vi "Supported Typedefs FGV.vi"() -> (3 "supported typedefs":set{string}(c389))   [LabVIEW 2020, in "MeasurementLink Measurement Server.lvlib"]
uses:
  MeasurementLink Measurement Server.lvlib
  gRPC/Generated APIs/ni/protobuf/types/RPC Messages/ni_protobuf_types_DoubleXYData.ctl
  gRPC/Generated APIs/ni/protobuf/types/ni.protobuf.types.lvlib
  <vilib>/Utility/Data Type/NI_Data Type.lvlib
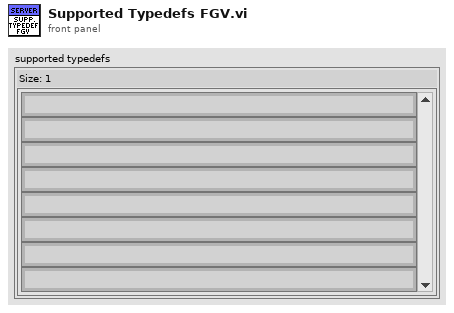
[diagram p1: front panel]
types:
  T1 = typedef "ni.protobuf.types.lvlib/ni_protobuf_types_DoubleXYData.ctl" = cluster{"x_data":dbl[], "y_data":dbl[]}
  T2 = typedef "NI_Data Type.lvlib/Type Definition Info.ctl" = cluster{"Name":string, "Timestamp":u32}
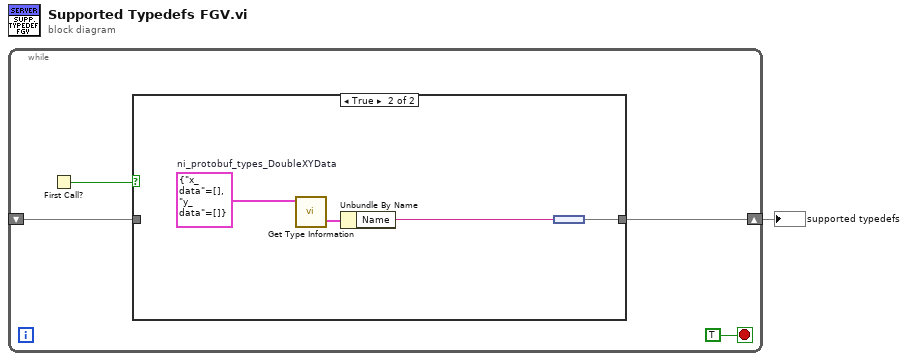
[diagram p0: block diagram]
diagram:
  n1 = while {
    shift-right: [w4] -> w1
    shift-left: _ -> [w3]
    stop <- TRUE stop-if-true
    n2 = First Call?() -> (First Call?: T/F=w5:bool)
    n3 = case shown="True" w5 {
      tunnel: [w6 w7] -> w4
      tunnel: w3 -> [w6 _]
      frame False {
      }
      frame True {
        w9 = T1 {"x_data"=[], "y_data"=[]}  # ni_protobuf_types_DoubleXYData
        n4 = call <vilib>:"Get Type Information.vi"("variant"=w9) -> ("type definition info"=w10:T2)  [unwired: 6 in, 4 out]
        n5 = Unbundle By Name(w10) -> ("Name"=w8:string)
        n6 = node(w8) -> (w7:set{string})
      }
    }
  }
  "supported typedefs" <- w1
